vi "initialize.vi"(4 "Tolerance (m)":dbl, 5 "Timeout (s)":dbl=-1.0, 6 "Duration (s)":dbl=-1.0, 7 "error in (no error)":errorcluster, 8 "Points of Interest":T1[](array[typedef]) {"North" format="%#_10f"; "East" format="%#_8f"}, 9 "Mission Type":T2=enum."Pass Between Buoys", 10 "RoundBouy in":refnum<class "RoundBouy.lvclass">) -> (0 "error out":errorcluster, 3 "RoundBouy out":refnum<class "RoundBouy.lvclass">)   [LabVIEW 2012, in "RoundBouy.lvclass"]
doc: "Round Bouy\nRequires:\na bouy location within an array\na rounding tolerance\nround left or round right enum"
uses:
  RoundBouy.lvclass
  Data/TypeDefs/MissionTypeControl.ctl
  Data/TypeDefs/UTM Location.ctl
  RoundBouy.lvclass/RoundBouy.ctl
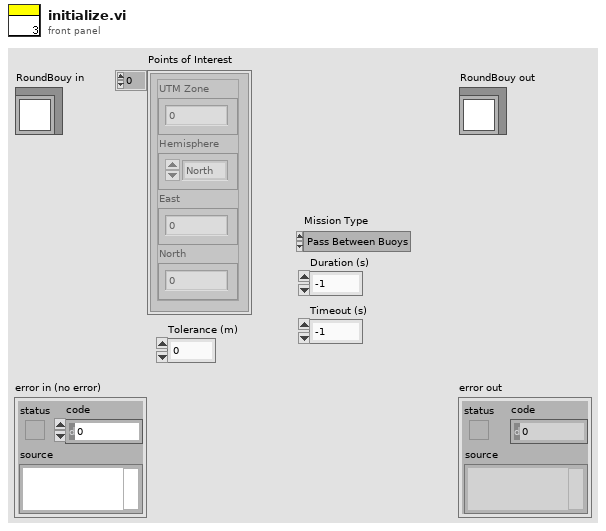
[diagram p1: front panel]
types:
  T1 = typedef "UTM Location.ctl" = cluster{"UTM Zone":dbl, "Hemisphere":enum16{"North", "South"}, "East":dbl, "North":dbl}
  T2 = typedef "MissionTypeControl.ctl" = enum16{"Idle at Point", "Drive to Waypoint", "Round Buoy to Port", "Round Buoy to Starboard", "Pass Between Buoys", "Station Keeping"}
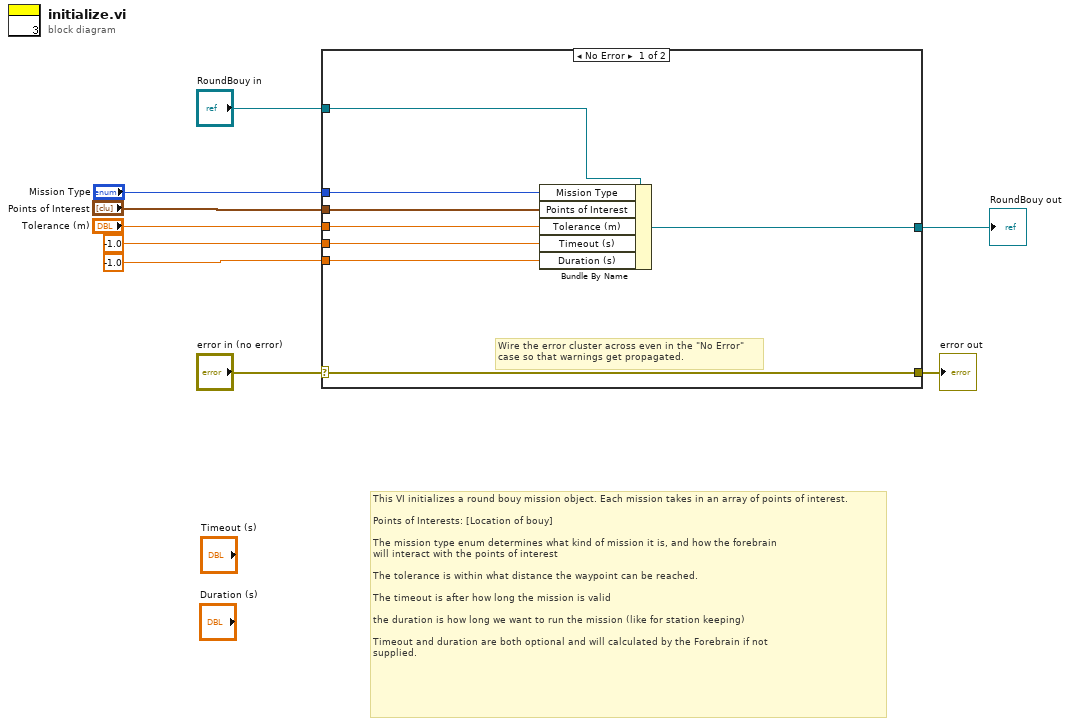
[diagram p0: block diagram]
diagram:
  # "This VI initializes a round bouy mission object. Each mission takes in an array of points of interest.\n\nPoints of Interests: [Location of bouy]\n\nThe mission type enum determines what kind of mission it is, and how the forebrain \nwill interact with the points of interest\n\nThe tolerance is within what distance the waypoint can be reached. \n\nThe timeout is after how long the mission is valid\n\nthe duration is how long we want to run the mission (like for station keeping)\n\nTimeout and duration are both optional and will calculated by the Forebrain if not \nsupplied."
  n1 = case shown="No Error" "error in (no error)" {
    selector: "error in (no error)" -> [w17 w19]
    tunnel: [w17 w19] -> w8
    tunnel: [w10 w18] -> w6
    tunnel: "RoundBouy in" -> [w16 w18]
    tunnel: "Points of Interest" -> [w15 _]
    tunnel: "Mission Type" -> [w14 _]
    tunnel: "Tolerance (m)" -> [w13 _]
    tunnel: -1.0 ("Timeout (s)") -> [w12 _]
    tunnel: -1.0 ("Duration (s)") -> [w11 _]
    frame No Error {
      # "Wire the error cluster across even in the \"No Error\"\ncase so that warnings get propagated."
      n2 = Bundle By Name(cluster=w16, "Mission Type"=w14, "Points of Interest"=w15, "Tolerance (m)"=w13, "Timeout (s)"=w12, "Duration (s)"=w11) -> (w10:refnum<class "RoundBouy.lvclass">)
    }
    frame Error {
    }
  }
  "error out" <- w8
  "RoundBouy out" <- w6
